vi "NGTS_Create Gain Schedule.vi"(8 "error in":errorcluster, 11 "tag_data_in":dbl[](array[numeric])) -> (0 "error out":errorcluster, 3 "PID gain schedule":T1(array[cluster])=[{"PID gains"={"proportional gain (Kc)"=1.0, "integral time (Ti, min)"=0.01, "derivative time (Td, min)"=0.0}, "max value"=100.0}] {"max value" format="%.2f"; "PID gains"."derivative time (Td, min)" format="%.3f"; "PID gains"."integral time (Ti, min)" format="%.3f"; "PID gains"."proportional gain (Kc)" format="%.3f"})   [LabVIEW 2010]
doc: "Accepts an array of doubles representing PID gain schedules in the order\n\n2007 Mike Ashe\nmichael.ashe@imaginatics.net\nCell: 860-961-0876"
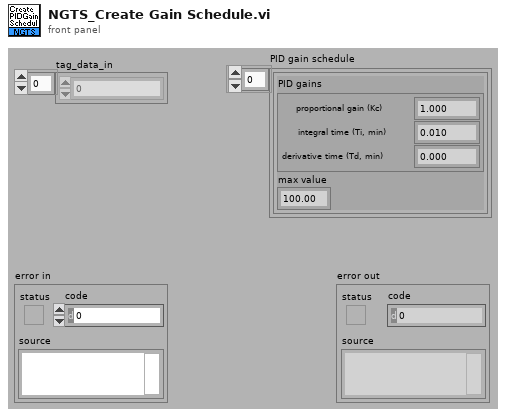
[diagram p1: front panel]
types:
  T1 = cluster{"PID gains":cluster{"proportional gain (Kc)":dbl, "integral time (Ti, min)":dbl, "derivative time (Td, min)":dbl}, "max value":dbl}[]
  T2 = cluster{"PID gains":cluster{"proportional gain (Kc)":dbl, "integral time (Ti, min)":dbl, "derivative time (Td, min)":dbl}, "max value":dbl}
  T3 = cluster{"Numeric":dbl, "Numeric":dbl, "Numeric":dbl}
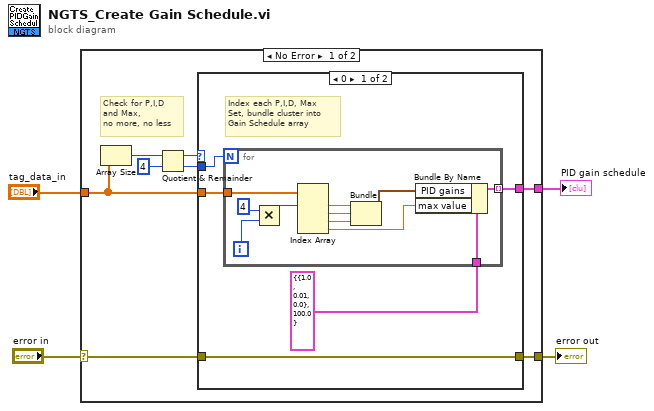
[diagram p0: block diagram]
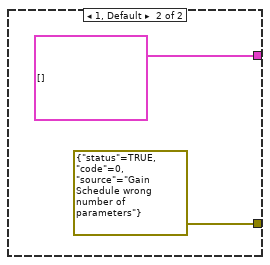
[diagram p2: hidden frame]
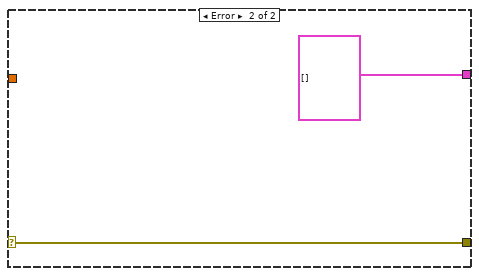
[diagram p3: hidden frame]
diagram:
  n1 = case shown="No Error" "error in" {
    selector: "error in" -> [w10 w31]
    tunnel: "tag_data_in" -> [w7 _]
    tunnel: [w6 T1 [] ("PID gain schedule")] -> w2
    tunnel: [w9 w31] -> w1
    frame No Error {
      # "Check for P,I,D\nand Max,\nno more, no less"
      n2 = Array Size(array=w7) -> (size(s)=w12:i32)
      n3 = Quotient & Remainder(x=w12, y=4) -> (x-y*floor(x/y)=w8:i32, floor(x/y)=w5:i32)
      n4 = case shown="0" w8 {
        tunnel: w10 -> [w17 _]
        tunnel: [w17 errorcluster {"status"=TRUE, "code"=0, "source"="Gain Schedule wrong number of parameters"} ("error IO")] -> w9
        tunnel: w7 -> [w16 _]
        tunnel: [w14 T1 [] ("PID gain schedule")] -> w6
        tunnel: w5 -> [w13 _]
        frame 0 {
          # "Index each P,I,D, Max\nSet, bundle cluster into\nGain Schedule array"
          n5 = for {
            N: w13 -> [_]
            tunnel: w16 -> [w28]
            tunnel: T2 {"PID gains"={"proportional gain (Kc)"=1.0, "integral time (Ti, min)"=0.01, "derivative time (Td, min)"=0.0}, "max value"=100.0} ("gain schedule") -> [w24]
            tunnel: [w18] -> w14 mode=indexing
            i -> [w27]
            n6 = Multiply(x=4 ("y"), y=w27) -> (x*y=w25:i32)
            n7 = Index Array(array=w28, index #1=w25) -> (element #1=w21:dbl, element #2=w22:dbl, element #3=w23:dbl, element #4=w19:dbl)  [unwired: 3 in]
            n8 = Bundle("Numeric"=w21, "Numeric"=w22, "Numeric"=w23) -> (w20:T3)  [unwired: 1 in]
            n9 = Bundle By Name(cluster=w24, "PID gains"=w20, "max value"=w19) -> (w18:T2)
          }
        }
        frame 1, Default {
        }
      }
    }
    frame Error {
    }
  }
  "PID gain schedule" <- w2
  "error out" <- w1
